vi "monochromatorCommandSetFilter.vi"(8 "error in":errorcluster, 10 "filter":i32, 11 "monochromator":refnum<k24>) -> (0 "error out":errorcluster, 3 "monochromator":refnum<k24>)   [LabVIEW 2009]
doc: "Set filter for monochromator"
uses:
  C:/Users/anderson.chen/Desktop/Software Development/Cornerstone Series API (LV9)/Cornerstone DLL/Cornerstone.dll
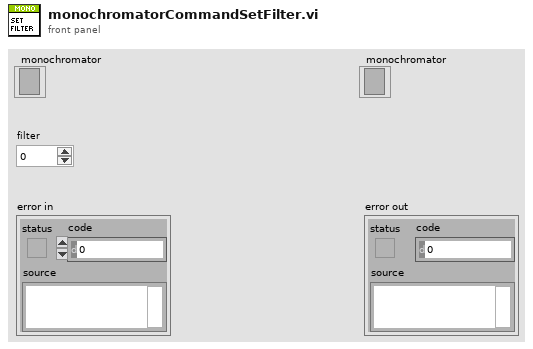
[diagram p1: front panel]
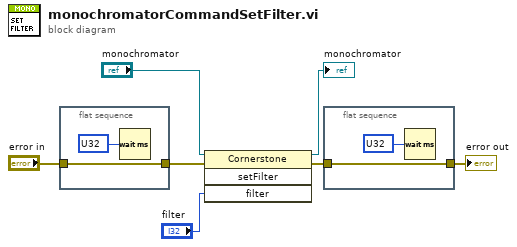
[diagram p0: block diagram]
diagram:
  n1 = flat-sequence {
    tunnel: "error in" -> [w8]
    tunnel: [w8] -> w3
    frame #0 {
      n2 = Wait (ms)(milliseconds to wait=u32 ?) -> ()  [unwired: 1 out]
    }
  }
  n3 = invoke class="Cornerstone" method="setFilter"(reference="monochromator", error in=w3, "filter"="filter") -> (reference out=→"monochromator":refnum<k24>, error out=w2:errorcluster)  [unwired: 1 in, 2 out]
  n4 = flat-sequence {
    tunnel: w2 -> [w10]
    tunnel: [w10] -> w1
    frame #0 {
      n5 = Wait (ms)(milliseconds to wait=u32 ?) -> ()  [unwired: 1 out]
    }
  }
  "error out" <- w1
